vi "Read Attributes.vi"(11 "Set Load Control Msg":refnum<class "Set Load Control Msg.lvclass">) -> (2 "Payload":cluster{"Load_Control":T1})   [LabVIEW 2018, in "Device Communication and Control Abstract Actor.lvlib" / "Set Load Control Msg.lvclass"]
uses:
  Set Load Control Msg.lvclass
  <vilib>/ORNL/CSEISMIC DDS/CSEISMIC DDS Base/Data Types/Load_Control.ctl
  <vilib>/ORNL/CSEISMIC DDS/CSEISMIC DDS Base/Data Types/Controls/DeviceID.ctl
  Set Load Control Msg.lvclass/Set Load Control Msg.ctl
  <vilib>/ORNL/CSEISMIC DDS/CSEISMIC DDS Base/CSEISMIC DDS.lvclass
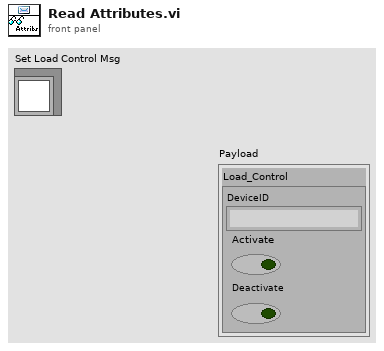
[diagram p1: front panel]
types:
  T1 = typedef "CSEISMIC DDS.lvlib/CSEISMIC DDS.lvclass/Load_Control.ctl" = cluster{"DeviceID":T2, "Activate":bool, "Deactivate":bool}
  T2 = typedef "CSEISMIC DDS.lvlib/CSEISMIC DDS.lvclass/DeviceID.ctl" = string
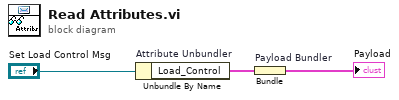
[diagram p0: block diagram]
diagram:
  n1 = Unbundle By Name "Attribute Unbundler"("Set Load Control Msg") -> ("Load_Control"=w1:T1)
  n2 = Bundle "Payload Bundler"("Load_Control"=w1) -> (→"Payload":cluster{"Load_Control":T1})  [unwired: 1 in]
